vi "BioFeedback8(8-channelSubViewTo2DVR).vi"(0 "UI Data Right":path=path "C:/Users/Tinggroup/Desktop/VRMuscleActivationVisualizer/VRBiofeedback_v2/assets/RightEMGData.txt", 7 "Frames Per Second":dbl=30.0, 9 "Start Trial":bool, 11 "End Trial":bool, 12 "Data Directory":path, 13 "File Name":string, 14 "Extension":string="_EMG.txt") -> ()   [LabVIEW 2016]
uses:
  <vilib>/Utility/error.llb/DialogType.ctl
  <vilib>/Analysis/5stat.llb/RMS (DBL).vi
  <vilib>/Waveform/WDTOps.llb/WDT Append Waveforms DBL.vi
  <vilib>/Waveform/WDTFileIO.llb/Export Waveform To Spreadsheet File.vi
  <vilib>/Analysis/NI_AALPro.lvlib
panel:
  in  "UI Ampl Error Path":path=path "C:/Users/Tinggroup/Desktop/VRMuscleActivationVisualizer/VRBiofeedback_v2/assets/BiofeedbackAmplitudeError.txt"
  in  "UI L/R Error Path":path=path "C:/Users/Tinggroup/Desktop/VRMuscleActivationVisualizer/VRBiofeedback_v2/assets/BiofeedbackLRError.txt"
  out "LeftPercentActivation":dbl
  out "RightPercentActivation":dbl
  out "LeftMovingAvg":dbl
  out "RightMovingAvg":dbl
  out "Stability Data":dbl[](array[numeric])
  in  "StabilityBufferFramesCount":dbl=1.0
  out "StabilityFramesCount":dbl
  in  "GuageStability":bool
  out "StdDev":dbl
  out "Mean":dbl
  out "Min":dbl
  out "Max":dbl
  in  "AutoAnalyzeStablity":bool
  out "RMS Left Single Bucket":dbl(graph)
  out "PointCluster":cluster{dbl[], dbl[]}
  out "combined y value":dbl
  out "Acquiring Max":bool
  in  "endGetMax":bool
  in  "startGetMax":bool
  in  "Right Max":dbl
  in  "Left Max":dbl
  in  "Amplitude Error":dbl
  in  "L/R error":dbl
  out "Target Graph":cluster{dbl[], dbl[]}[](graph)
  in  "RightSignalB":dbl=6.0
  in  "RightSignalA":dbl=5.0
  in  "LefftSignalB":dbl=2.0
  in  "LeftSignalA":dbl=1.0
  out "Aggregate 8":waveform(dbl)[](array[waveform])
  in  "UI Data Left":path=path "C:/Users/Tinggroup/Desktop/VRMuscleActivationVisualizer/VRBiofeedback_v2/assets/LeftEMGData.txt"
  in  "EMG Input Device\nProduct Type":string="USB-6009"
  out "DispLeftMovingAvg":dbl(slide) max=1.0 scale=0.0..100.0
  out "DispRightMovingAvg":dbl(slide) max=0.01 scale=0.0..100.0
  out "RMS Right":dbl(graph)
  out "RMS Left":dbl(graph)
  out "RMS 8":dbl(graph)
  out "RMS 7":dbl(graph)
  out "RMS 6":dbl(graph)
  out "RMS 5":dbl(graph)
  out "RMS 4":dbl(graph)
  out "RMS 3":dbl(graph)
  out "RMS 2":dbl(graph)
  out "RMS 1":dbl(graph)
  out "Aggregate7":waveform(dbl)[](array[waveform])
  out "Aggregate6":waveform(dbl)[](array[waveform])
  out "Aggregate5":waveform(dbl)[](array[waveform])
  out "Aggregate4":waveform(dbl)[](array[waveform])
  out "Aggregate3":waveform(dbl)[](array[waveform])
  out "Aggregate2":waveform(dbl)[](array[waveform])
  out "Aggregate1":waveform(dbl)[](array[waveform])
  out "Wfm8":waveform(dbl)(graph)
  out "Wfm7":waveform(dbl)(graph)
  out "Wfm6":waveform(dbl)(graph)
  out "Wfm5":waveform(dbl)(graph)
  out "Wfm4":waveform(dbl)(graph)
  out "Wfm3":waveform(dbl)(graph)
  out "Wfm2":waveform(dbl)(graph)
  out "Wfm1":waveform(dbl)(graph)
  out "Trial Data":waveform(dbl)(graph)
  in  "UI Percent Path":path=path "C:/Users/Tinggroup/Desktop/VRMuscleActivationVisualizer/VRBiofeedback_v2/assets/BiofeedbackTargetPercentage.txt"
  in  "Target Percentage":dbl=10.0
  out "Trial In Progress":bool
  in  "Trial Number":dbl
  in  "MARK":bool
  in  "Lower Cut-Off":dbl=20.0
  in  "Upper Cut-Off":dbl=300.0
  out "raw data":dynamicdata(graph)
  out "Bufffer Index":dbl
  out "Frames in Buffer":dbl
  out "Samples per frame":dbl
  out "Reset Data Acquisition\nAnd UI Updating":bool=TRUE
  in  "Moving Average Length (s)":dbl=0.5
  in  "Sample rate (Hz)":dbl=2000.0
  in  "End Program":bool
  # "These \nSet \nThe \nTarget\nBox Size"
  # "Save Trial Data"
  # "These scale\nthe thermometers\nand are used in\nmean calculation"
  # "Auto Analyze Stability begins calculating stability\nAs soon as dot enters the target zone and stops \nonce the dot leaves the target zone"
  # "for testing smaller sample\nsizes in getting max/min\nand stability data"
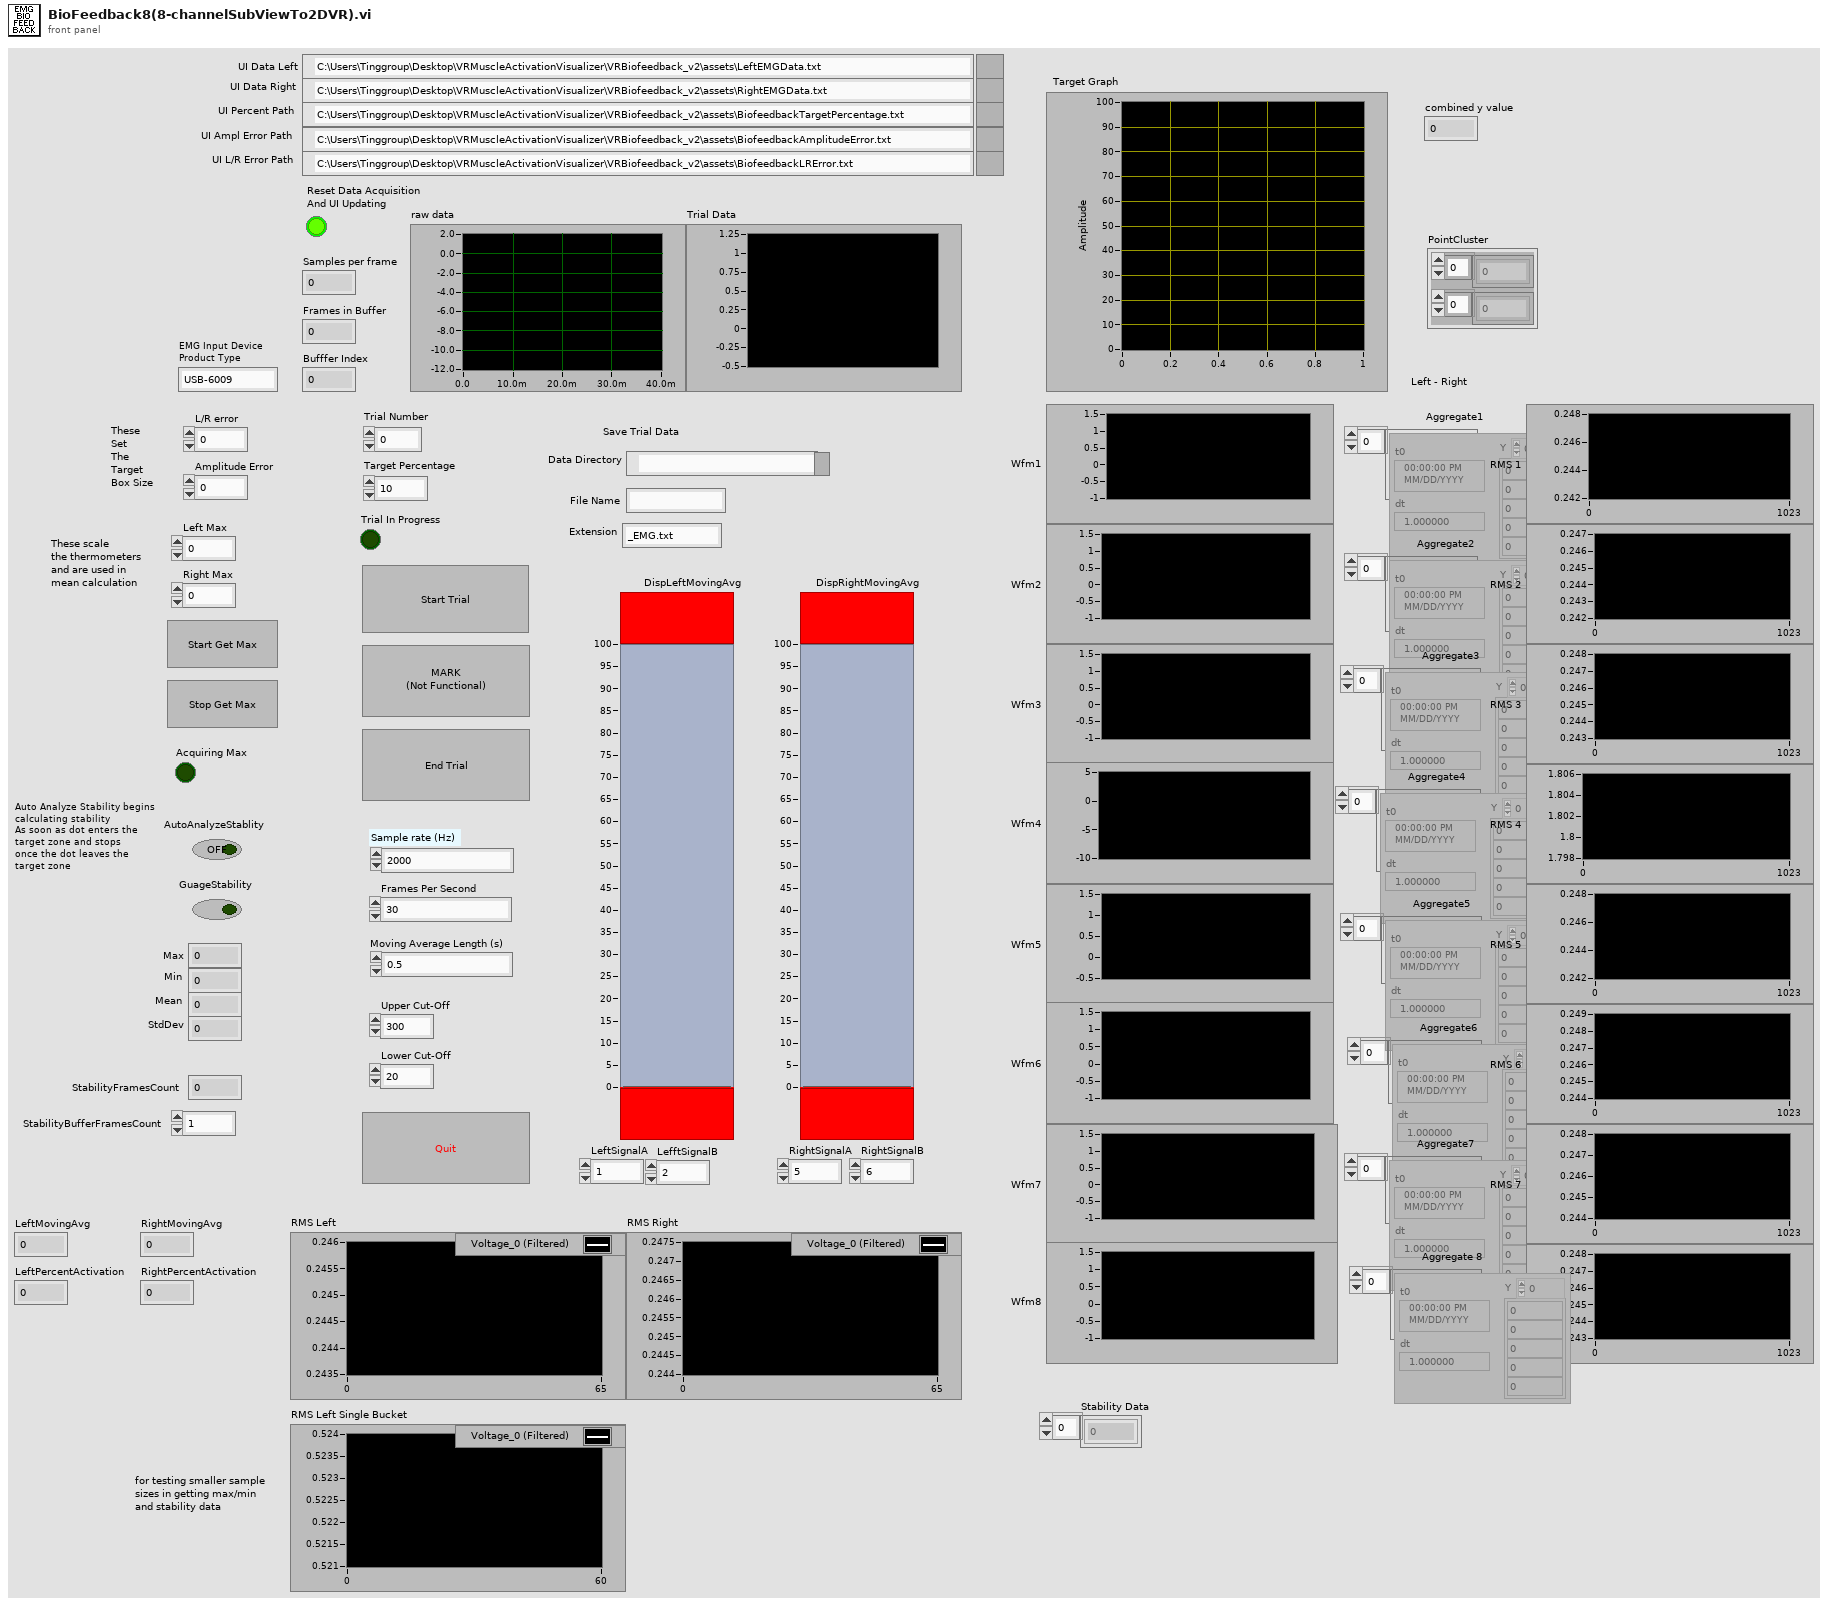
[diagram p1: front panel]
types:
  T1 = typedef "DialogType.ctl" = u16
  T2 = typedef "WaveformArrayControl.ctl" = waveform(dbl)[]
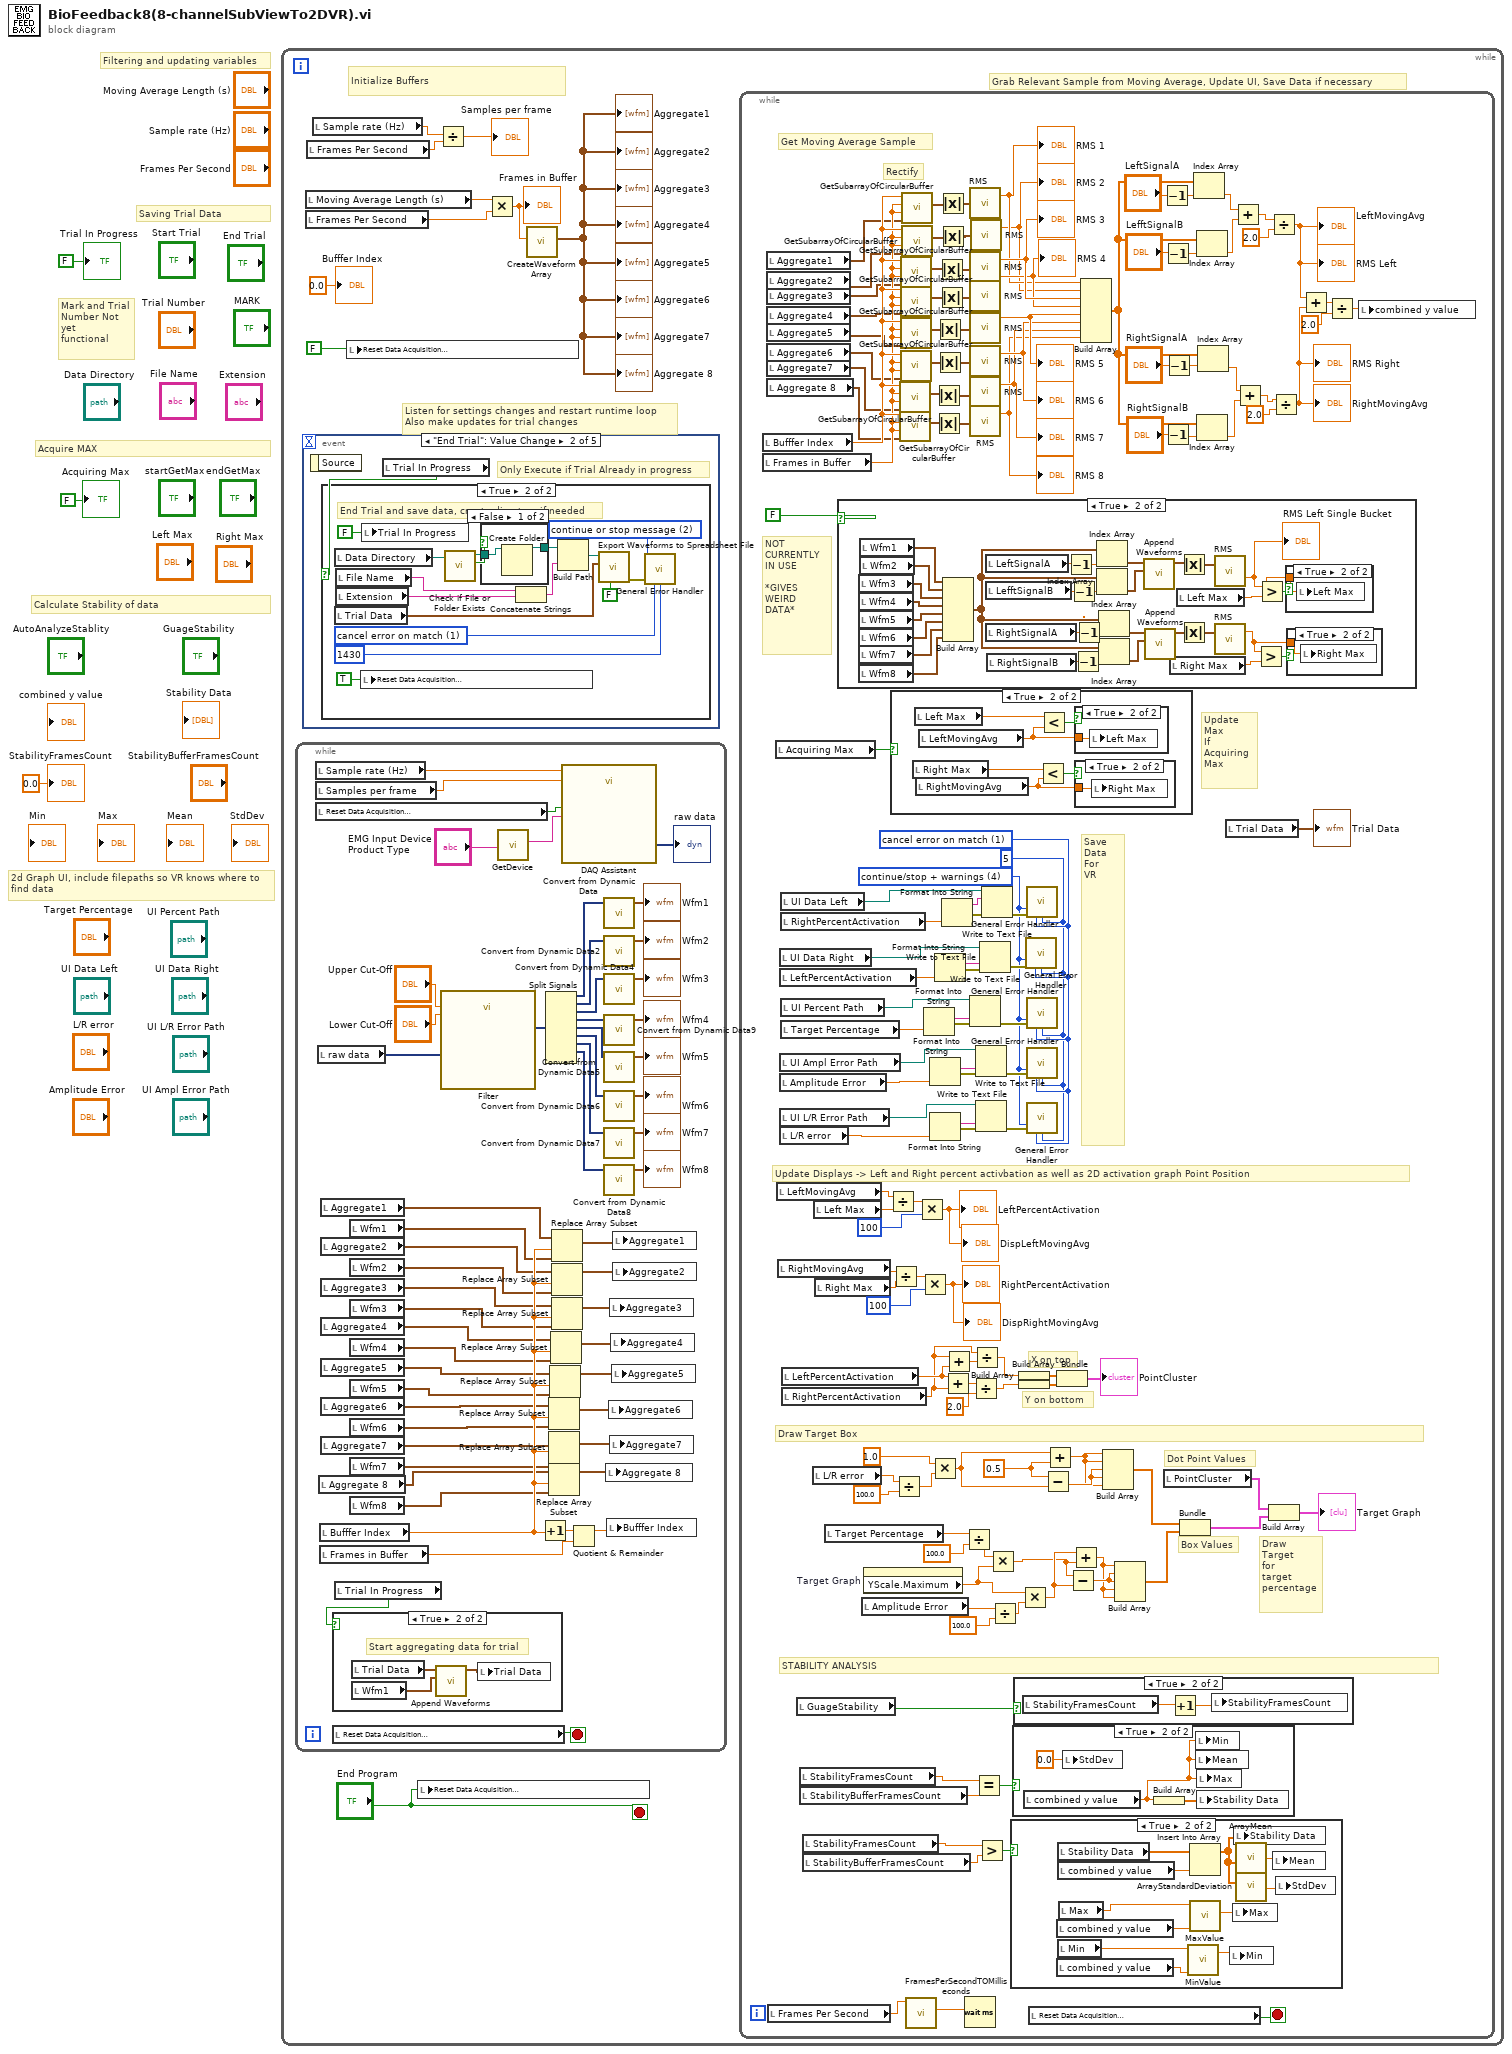
[diagram p0: block diagram]
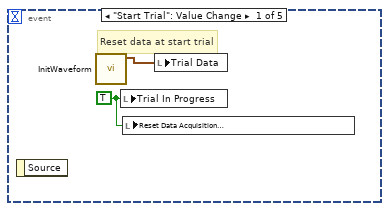
[diagram p2: hidden frame]
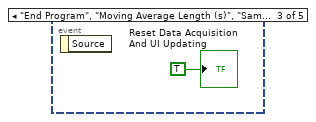
[diagram p5: hidden frame]
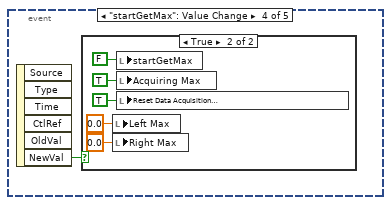
[diagram p6: hidden frame]
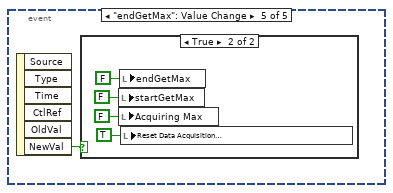
[diagram p8: hidden frame]
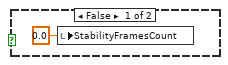
[diagram p12: hidden frame]
diagram:
  # "Calculate Stability of data"
  # "Acquire MAX"
  # "Filtering and updating variables"
  # "Saving Trial Data"
  # "2d Graph UI, include filepaths so VR knows where to find data"
  # "Mark and Trial Number Not yet \nfunctional"
  n1 = while {
    stop <- "End Program" stop-if-true
    # "Grab Relevant Sample from Moving Average, Update UI, Save Data if necessary"
    # "Initialize Buffers"
    # "Listen for settings changes and restart runtime loop\nAlso make updates for trial changes"
    n2 = while {
      stop <- w294 stop-if-true
      n3 = local read "Sample rate (Hz)"() -> (w302:dbl)
      n4 = local read "Samples per frame"() -> (w301:dbl)
      n5 = local read "Reset Data Acquisition\nAnd UI Updating"() -> (w293:bool)
      n6 = local read "raw data"() -> (w299:dynamicdata)
      n7 = local read "Aggregate 8"() -> (w249:waveform(dbl)[])
      n8 = local read "Bufffer Index"() -> (w274:dbl)
      n9 = local read "Frames in Buffer"() -> (w296:dbl)
      n10 = local read "Aggregate1"() -> (w273:waveform(dbl)[])
      n11 = local read "Aggregate2"() -> (w271:waveform(dbl)[])
      n12 = local read "Aggregate3"() -> (w269:waveform(dbl)[])
      n13 = local read "Aggregate4"() -> (w267:waveform(dbl)[])
      n14 = local read "Aggregate5"() -> (w265:waveform(dbl)[])
      n15 = local read "Aggregate6"() -> (w263:waveform(dbl)[])
      n16 = local read "Aggregate7"() -> (w261:waveform(dbl)[])
      n17 = local read "Reset Data Acquisition\nAnd UI Updating"() -> (w294:bool)
      n18 = local read "Trial In Progress"() -> (w251:bool)
      n19 = case shown="True" w251 {
        frame False {
        }
        frame True {
          # "Start aggregating data for trial"
          n20 = local read "Trial Data"() -> (w305:waveform(dbl))
          n21 = local read "Wfm1"() -> (w304:waveform(dbl))
          n22 = call-poly <vilib>:"Append Waveforms.vi"("waveform B"=w304, "waveform A"=w305) -> ("waveform out"=w303:waveform(dbl))  [unwired: 8 in, 1 out]
          n23 = local write "Trial Data"(w303) -> ()
        }
      }
      n24 = local read "Wfm1"() -> (w272:waveform(dbl))
      n25 = local read "Wfm2"() -> (w270:waveform(dbl))
      n26 = local read "Wfm3"() -> (w268:waveform(dbl))
      n27 = local read "Wfm4"() -> (w266:waveform(dbl))
      n28 = local read "Wfm5"() -> (w264:waveform(dbl))
      n29 = local read "Wfm6"() -> (w262:waveform(dbl))
      n30 = local read "Wfm7"() -> (w260:waveform(dbl))
      n31 = local read "Wfm8"() -> (w259:waveform(dbl))
      n32 = call "Filter"("Lower Cut-Off"="Lower Cut-Off", "Upper Cut-Off"="Upper Cut-Off", "Signal"=w299) -> ("Filtered Signal"=w291:dynamicdata)  [unwired: 7 in, 1 out]
      n33 = call "GetDevice.vi"("EMG Input Device\nProduct Type"="EMG Input Device\nProduct Type") -> ("DAQmx Device Name"=w247:tag)  [unwired: 10 in]
      n34 = Increment(x=w274) -> (x+1=w295:dbl)
      n35 = Split Signals(w291) -> (w290:dynamicdata, w289:dynamicdata, w288:dynamicdata, w287:dynamicdata, w286:dynamicdata, w285:dynamicdata, w284:dynamicdata, w283:dynamicdata)  [unwired: 9 in, 1 out]
      n36 = Replace Array Subset(array=w263, new element=w262, index=w274) -> (w253:waveform(dbl)[])
      n37 = Replace Array Subset(array=w261, new element=w260, index=w274) -> (w252:waveform(dbl)[])
      n38 = Replace Array Subset(array=w249, new element=w259, index=w274) -> (w250:waveform(dbl)[])
      n39 = Replace Array Subset(array=w265, new element=w264, index=w274) -> (w254:waveform(dbl)[])
      n40 = Replace Array Subset(array=w267, new element=w266, index=w274) -> (w255:waveform(dbl)[])
      n41 = Replace Array Subset(array=w273, new element=w272, index=w274) -> (w258:waveform(dbl)[])
      n42 = Replace Array Subset(array=w271, new element=w270, index=w274) -> (w257:waveform(dbl)[])
      n43 = Replace Array Subset(array=w269, new element=w268, index=w274) -> (w256:waveform(dbl)[])
      n44 = call "DAQ Assistant"("rate"=w302, "number of samples"=w301, "stop (T)"=w293, "device name"=w247) -> ("data"=→"raw data":dynamicdata)  [unwired: 13 in, 2 out]
      n45 = Quotient & Remainder(x=w295, y=w296) -> (x-y*floor(x/y)=w297:dbl)  [unwired: 1 out]
      n46 = call "Convert from Dynamic Data"("Dynamic Data Type"=w290) -> ("Waveform"=→"Wfm1":waveform(dbl))  [unwired: 3 in]
      n47 = call "Convert from Dynamic Data2"("Dynamic Data Type"=w289) -> ("Waveform"=→"Wfm2":waveform(dbl))  [unwired: 3 in]
      n48 = call "Convert from Dynamic Data4"("Dynamic Data Type"=w288) -> ("Waveform"=→"Wfm3":waveform(dbl))  [unwired: 3 in]
      n49 = call "Convert from Dynamic Data9"("Dynamic Data Type"=w287) -> ("Waveform"=→"Wfm4":waveform(dbl))  [unwired: 3 in]
      n50 = call "Convert from Dynamic Data5"("Dynamic Data Type"=w286) -> ("Waveform"=→"Wfm5":waveform(dbl))  [unwired: 3 in]
      n51 = call "Convert from Dynamic Data6"("Dynamic Data Type"=w285) -> ("Waveform"=→"Wfm6":waveform(dbl))  [unwired: 3 in]
      n52 = call "Convert from Dynamic Data7"("Dynamic Data Type"=w284) -> ("Waveform"=→"Wfm7":waveform(dbl))  [unwired: 3 in]
      n53 = call "Convert from Dynamic Data8"("Dynamic Data Type"=w283) -> ("Waveform"=→"Wfm8":waveform(dbl))  [unwired: 3 in]
      n54 = local write "Aggregate 8"(w250) -> ()
      n55 = local write "Bufffer Index"(w297) -> ()
      n56 = local write "Aggregate6"(w253) -> ()
      n57 = local write "Aggregate3"(w256) -> ()
      n58 = local write "Aggregate7"(w252) -> ()
      n59 = local write "Aggregate4"(w255) -> ()
      n60 = local write "Aggregate5"(w254) -> ()
      n61 = local write "Aggregate1"(w258) -> ()
      n62 = local write "Aggregate2"(w257) -> ()
    }
    n63 = event shown="[1] \"End Trial\": Value Change" {
      selector: _ -> [_ _ _ _ _]
      dyn-events: _ -> [_ _ _ _ _]
      timeout: _ -> [_ _ _ _ _]
      event "Start Trial": Value Change {
        w14 = TRUE ("Trial In Progress")
        # "Reset data at start trial"
        n64 = event-data() -> ()  [unwired: 1 in, 1 out]
        n65 = call "InitWaveform.vi"() -> ("output waveform"=w15:waveform(dbl))  [unwired: 11 in]
        n66 = local write "Trial In Progress"(w14) -> ()
        n67 = local write "Reset Data Acquisition\nAnd UI Updating"(w14) -> ()
        n68 = local write "Trial Data"(w15) -> ()
      }
      event "End Trial": Value Change {
        # "Only Execute if Trial Already in progress"
        n69 = event-data() -> ()  [unwired: 1 in, 1 out]
        n70 = local read "Trial In Progress"() -> (w16:bool)
        n71 = case shown="True" w16 {
          frame False {
          }
          frame True {
            w25 = T1 2 items=["no dialog", "OK message", "continue or stop message", "OK message + warnings", "continue/stop + warnings"] ("type of dialog (OK msg:1)")
            w26 = 1 items=["no exception", "cancel error on match", "set error on match"] ("[exception action] (none:0)")
            # "End Trial and save data, create directory if needed"
            n72 = local read "Data Directory"() -> (w28:path)
            n73 = local read "Trial Data"() -> (w18:waveform(dbl))
            n74 = local read "File Name"() -> (w20:string)
            n75 = local read "Extension"() -> (w21:string)
            n76 = local write "Reset Data Acquisition\nAnd UI Updating"(TRUE ("Reset Data Acquisition\nAnd UI Updating")) -> ()
            n77 = local write "Trial In Progress"(FALSE ("Trial In Progress")) -> ()
            n78 = call <vilib>:"Check if File or Folder Exists.vi"("path"=w28) -> ("file or folder exists?"=w30:bool, "dup path"=w29:path)  [unwired: 8 in, 1 out]
            n79 = case shown="False" w30 {
              tunnel: [w33 w35] -> w24
              tunnel: w29 -> [w34 w35]
              frame False {
                n80 = Create Folder(path (use dialog)=w34) -> (created path=w33:path)  [unwired: 2 in, 2 out]
              }
              frame True {
              }
            }
            n81 = Concatenate Strings(w20, w21) -> (w19:string)
            n82 = Build Path(base path=w24, name or relative path=w19) -> (appended path=w23:path)
            n83 = call-poly <vilib>:"Export Waveforms to Spreadsheet File.vi"("append to file? (new file:F)"=FALSE, "waveform"=w18, "file path (dialog if empty)"=w23) -> ("error out"=w17:errorcluster)  [unwired: 7 in, 1 out]
            n84 = call <vilib>:"General Error Handler.vi"("type of dialog (OK msg:1)"=w25, "error in (no error)"=w17, "[exception action] (none:0)"=w26, "[exception code]"=1430) -> ()  [unwired: 7 in, 5 out]
          }
        }
      }
      event "End Program", "Moving Average Length (s)", "Sample rate (Hz)", "Frames Per Second": Value Change {
        n85 = event-data() -> ()  [unwired: 1 in, 1 out]
        "Reset Data Acquisition\nAnd UI Updating" <- TRUE
      }
      event "startGetMax": Value Change {
        n86 = event-data() -> ("NewVal"=w37:bool)  [unwired: 1 in, 5 out]
        n87 = case shown="True" w37 {
          frame False {
          }
          frame True {
            n88 = local write "Left Max"(0.0 ("Left Max")) -> ()
            n89 = local write "Right Max"(0.0 ("Right Max")) -> ()
            n90 = local write "startGetMax"(FALSE) -> ()
            n91 = local write "Acquiring Max"(TRUE ("Acquiring Max")) -> ()
            n92 = local write "Reset Data Acquisition\nAnd UI Updating"(TRUE ("Reset Data Acquisition\nAnd UI Updating")) -> ()
          }
        }
      }
      event "endGetMax": Value Change {
        n93 = event-data() -> ("NewVal"=w43:bool)  [unwired: 1 in, 5 out]
        n94 = case shown="True" w43 {
          frame False {
          }
          frame True {
            n95 = local write "startGetMax"(FALSE ("startGetMax")) -> ()
            n96 = local write "Acquiring Max"(FALSE ("Acquiring Max")) -> ()
            n97 = local write "endGetMax"(FALSE ("endGetMax")) -> ()
            n98 = local write "Reset Data Acquisition\nAnd UI Updating"(TRUE ("Reset Data Acquisition\nAnd UI Updating")) -> ()
          }
        }
      }
    }
    n99 = local read "Moving Average Length (s)"() -> (w10:dbl)
    n100 = local read "Frames Per Second"() -> (w9:dbl)
    n101 = local read "Frames Per Second"() -> (w12:dbl)
    n102 = local read "Sample rate (Hz)"() -> (w13:dbl)
    n103 = local write "Reset Data Acquisition\nAnd UI Updating"(FALSE) -> ()
    n104 = local write "Reset Data Acquisition\nAnd UI Updating"("End Program") -> ()
    n105 = Divide(x=w13, y=w12) -> (x/y=→"Samples per frame":dbl)
    n106 = Multiply(x=w10, y=w9) -> (x*y=w6:dbl)
    "Frames in Buffer" <- w6
    n107 = call "CreateWaveformArray.vi"("bufferSize"=w6) -> ("initialized array"=→"Aggregate1" →"Aggregate2" →"Aggregate3" →"Aggregate4" →"Aggregate5" →"Aggregate6" →"Aggregate7" →"Aggregate 8":waveform(dbl)[])  [unwired: 5 in, 1 out]
    n108 = while {
      stop <- w188 stop-if-true
      w106 = 0.5 ("element")
      w50 = T1 4 items=["no dialog", "OK message", "continue or stop message", "OK message + warnings", "continue/stop + warnings"] ("type of dialog (OK msg:1)")
      w49 = 1 items=["no exception", "cancel error on match", "set error on match"] ("[exception action] (none:0)")
      w48 = 5 ("[exception code]")
      # "Y on bottom"
      # "X on top"
      # "Dot Point Values"
      # "Box Values"
      # "Update Displays -> Left and Right percent activbation as well as 2D activation graph Point Position"
      # "STABILITY ANALYSIS"
      # "NOT\nCURRENTLY\nIN USE\n\n*GIVES\nWEIRD\nDATA*"
      # "Draw \nTarget\nfor\ntarget\npercentage"
      # "Draw Target Box"
      # "Update\nMax\nIf \nAcquiring\nMax"
      # "Save\nData\nFor\nVR"
      # "Get Moving Average Sample"
      # "Rectify"
      n109 = local read "Bufffer Index"() -> (w179:dbl)
      n110 = local read "Frames in Buffer"() -> (w178:dbl)
      n111 = local read "Aggregate1"() -> (w177:waveform(dbl)[])
      n112 = local read "Aggregate2"() -> (w173:waveform(dbl)[])
      n113 = local read "Aggregate3"() -> (w176:waveform(dbl)[])
      n114 = local read "Aggregate4"() -> (w172:waveform(dbl)[])
      n115 = local read "Aggregate5"() -> (w175:waveform(dbl)[])
      n116 = local read "Aggregate6"() -> (w174:waveform(dbl)[])
      n117 = local read "Aggregate7"() -> (w171:waveform(dbl)[])
      n118 = local read "Aggregate 8"() -> (w145:waveform(dbl)[])
      n119 = local read "Frames Per Second"() -> (w187:dbl)
      n120 = local read "Acquiring Max"() -> (w90:bool)
      n121 = local read "LeftMovingAvg"() -> (w79:dbl)
      n122 = local read "RightMovingAvg"() -> (w75:dbl)
      n123 = local read "UI Data Right"() -> (w183:path)
      n124 = local read "LeftPercentActivation"() -> (w181:dbl)
      n125 = local read "UI Ampl Error Path"() -> (w51:path)
      n126 = local read "Amplitude Error"() -> (w52:dbl)
      n127 = local read "UI L/R Error Path"() -> (w54:path)
      n128 = local read "L/R error"() -> (w53:dbl)
      n129 = local read "UI Data Left"() -> (w153:path)
      n130 = local read "RightPercentActivation"() -> (w155:dbl)
      n131 = local read "UI Percent Path"() -> (w147:path)
      n132 = local read "Target Percentage"() -> (w146:dbl)
      n133 = local read "LeftPercentActivation"() -> (w68:dbl)
      n134 = local read "RightPercentActivation"() -> (w66:dbl)
      n135 = local read "GuageStability"() -> (w88:bool)
      n136 = local read "StabilityFramesCount"() -> (w87:dbl)
      n137 = local read "StabilityBufferFramesCount"() -> (w86:dbl)
      n138 = local read "StabilityFramesCount"() -> (w84:dbl)
      n139 = local read "StabilityBufferFramesCount"() -> (w83:dbl)
      n140 = local read "L/R error"() -> (w125:dbl)
      n141 = local read "Left Max"() -> (w78:dbl)
      n142 = local read "Right Max"() -> (w74:dbl)
      n143 = local read "Target Percentage"() -> (w122:dbl)
      n144 = case shown="True" FALSE {
        frame False {
        }
        frame True {
          n145 = local read "Wfm3"() -> (w237:waveform(dbl))
          n146 = local read "Wfm4"() -> (w236:waveform(dbl))
          n147 = local read "Wfm5"() -> (w240:waveform(dbl))
          n148 = local read "Wfm6"() -> (w241:waveform(dbl))
          n149 = local read "Wfm7"() -> (w242:waveform(dbl))
          n150 = local read "Wfm8"() -> (w243:waveform(dbl))
          n151 = local read "Wfm1"() -> (w239:waveform(dbl))
          n152 = local read "Wfm2"() -> (w238:waveform(dbl))
          n153 = Build Array(w239, w238, w237, w236, w240, w241, w242, w243) -> (w235:waveform(dbl)[])
          n154 = local read "LeftSignalA"() -> (w221:dbl)
          n155 = local read "LefftSignalB"() -> (w219:dbl)
          n156 = local read "RightSignalA"() -> (w217:dbl)
          n157 = local read "RightSignalB"() -> (w214:dbl)
          n158 = Decrement(x=w221) -> (x-1=w220:dbl)
          n159 = Decrement(x=w219) -> (x-1=w218:dbl)
          n160 = Decrement(x=w214) -> (x-1=w215:dbl)
          n161 = Decrement(x=w217) -> (x-1=w216:dbl)
          n162 = Index Array(array=w235, index=w220) -> (element=w222:waveform(dbl))
          n163 = Index Array(array=w235, index=w218) -> (element=w223:waveform(dbl))
          n164 = Index Array(array=w235, index=w216) -> (element=w234:waveform(dbl))
          n165 = Index Array(array=w235, index=w215) -> (element=w233:waveform(dbl))
          n166 = call-poly <vilib>:"Append Waveforms.vi"("waveform B"=w223, "waveform A"=w222) -> ("waveform out"=w229:waveform(dbl))  [unwired: 8 in, 1 out]
          n167 = call-poly <vilib>:"Append Waveforms.vi"("waveform B"=w233, "waveform A"=w234) -> ("waveform out"=w232:waveform(dbl))  [unwired: 8 in, 1 out]
          n168 = local read "Right Max"() -> (w228:dbl)
          n169 = local read "Left Max"() -> (w244:dbl)
          n170 = Absolute Value(x=w229) -> (abs(x)=w230:waveform(dbl))
          n171 = Absolute Value(x=w232) -> (abs(x)=w231:waveform(dbl))
          n172 = call-poly <vilib>:"RMS.vi"("X"=w230) -> ("rms value"=w224:dbl)  [unwired: 1 out]
          "RMS Left Single Bucket" <- w224
          n173 = call-poly <vilib>:"RMS.vi"("X"=w231) -> ("rms value"=w227:dbl)  [unwired: 1 out]
          n174 = Greater?(x=w227, y=w228) -> (0:w226:bool)
          n175 = Greater?(x=w224, y=w244) -> (0:w225:bool)
          n176 = case shown="True" w225 {
            tunnel: w224 -> [_ w246]
            frame False {
            }
            frame True {
              n177 = local write "Left Max"(w246) -> ()
            }
          }
          n178 = case shown="True" w226 {
            tunnel: w227 -> [_ w245]
            frame False {
            }
            frame True {
              n179 = local write "Right Max"(w245) -> ()
            }
          }
        }
      }
      n180 = local read "Amplitude Error"() -> (w124:dbl)
      n181 = property on="Target Graph" class="XYGraph (strict)"() -> ("YScale.Maximum"=w104:dbl)  [unwired: 2 in, 2 out]
      n182 = Divide(x=w79, y=w78) -> (x/y=w80:dbl)
      n183 = case shown="True" w90 {
        frame False {
        }
        frame True {
          n184 = local read "Right Max"() -> (w208:dbl)
          n185 = local read "Left Max"() -> (w211:dbl)
          n186 = local read "RightMovingAvg"() -> (w206:dbl)
          n187 = local read "LeftMovingAvg"() -> (w210:dbl)
          n188 = Less?(x=w208, y=w206) -> (x < y?=w207:bool)
          n189 = Less?(x=w211, y=w210) -> (x < y?=w209:bool)
          n190 = case shown="True" w209 {
            tunnel: w210 -> [_ w213]
            frame False {
            }
            frame True {
              n191 = local write "Left Max"(w213) -> ()
            }
          }
          n192 = case shown="True" w207 {
            tunnel: w206 -> [_ w212]
            frame False {
            }
            frame True {
              n193 = local write "Right Max"(w212) -> ()
            }
          }
        }
      }
      n194 = Divide(x=w75, y=w74) -> (x/y=w76:dbl)
      n195 = Divide(x=w125, y=100.0) -> (x/y=w114:dbl)
      n196 = call "GetSubarrayOfCircularBuffer.vi"("initialized array"=w171, "buffer size"=w178, "subset size"=w178, "start index"=w179) -> ("initialized array 2"=w164:T2)  [unwired: 7 in]
      n197 = call "GetSubarrayOfCircularBuffer.vi"("initialized array"=w145, "buffer size"=w178, "subset size"=w178, "start index"=w179) -> ("initialized array 2"=w163:T2)  [unwired: 7 in]
      n198 = call "GetSubarrayOfCircularBuffer.vi"("initialized array"=w176, "buffer size"=w178, "subset size"=w178, "start index"=w179) -> ("initialized array 2"=w168:T2)  [unwired: 7 in]
      n199 = call "GetSubarrayOfCircularBuffer.vi"("initialized array"=w172, "buffer size"=w178, "subset size"=w178, "start index"=w179) -> ("initialized array 2"=w167:T2)  [unwired: 7 in]
      n200 = call "GetSubarrayOfCircularBuffer.vi"("initialized array"=w175, "buffer size"=w178, "subset size"=w178, "start index"=w179) -> ("initialized array 2"=w166:T2)  [unwired: 7 in]
      n201 = call "GetSubarrayOfCircularBuffer.vi"("initialized array"=w174, "buffer size"=w178, "subset size"=w178, "start index"=w179) -> ("initialized array 2"=w165:T2)  [unwired: 7 in]
      n202 = call "GetSubarrayOfCircularBuffer.vi"("initialized array"=w177, "buffer size"=w178, "subset size"=w178, "start index"=w179) -> ("initialized array 2"=w170:T2)  [unwired: 7 in]
      n203 = call "GetSubarrayOfCircularBuffer.vi"("initialized array"=w173, "buffer size"=w178, "subset size"=w178, "start index"=w179) -> ("initialized array 2"=w169:T2)  [unwired: 7 in]
      n204 = call "FramesPerSecondTOMilliseconds.vi"("Thermometer\nFps"=w187) -> ("x*y"=w186:dbl)  [unwired: 10 in]
      n205 = Multiply(x=w80, y=100) -> (x*y=→"DispLeftMovingAvg" →"LeftPercentActivation":dbl)
      n206 = Multiply(x=w76, y=100) -> (x*y=→"DispRightMovingAvg" →"RightPercentActivation":dbl)
      n207 = Format Into String(w146) -> (resulting string=w148:string, error out=w149:errorcluster)  [unwired: 3 in]
      n208 = Format Into String(w52) -> (resulting string=w58:string, error out=w59:errorcluster)  [unwired: 3 in]
      n209 = Format Into String(w53) -> (resulting string=w55:string, error out=w56:errorcluster)  [unwired: 3 in]
      n210 = Multiply(x=1.0, y=w114) -> (x*y=w113:dbl)
      n211 = Absolute Value(x=w164) -> (abs(x)=w157:T2)
      n212 = Absolute Value(x=w163) -> (abs(x)=w156:T2)
      n213 = Absolute Value(x=w166) -> (abs(x)=w159:T2)
      n214 = Absolute Value(x=w165) -> (abs(x)=w158:T2)
      n215 = Format Into String(w181) -> (resulting string=w182:string, error out=w184:errorcluster)  [unwired: 3 in]
      n216 = Absolute Value(x=w168) -> (abs(x)=w161:T2)
      n217 = Absolute Value(x=w167) -> (abs(x)=w160:T2)
      n218 = Absolute Value(x=w170) -> (abs(x)=w162:T2)
      n219 = Absolute Value(x=w169) -> (abs(x)=w144:T2)
      n220 = Format Into String(w155) -> (resulting string=w152:string, error out=w154:errorcluster)  [unwired: 3 in]
      n221 = Add(x=w68, y=w66) -> (x+y=w70:dbl)
      n222 = Add(x=w66, y=w68) -> (x+y=w67:dbl)
      n223 = Divide(x=w122, y=100.0) -> (x/y=w105:dbl)
      n224 = Wait (ms)(milliseconds to wait=w186) -> ()  [unwired: 1 out]
      n225 = call-poly <vilib>:"RMS.vi"("X"=w162) -> ("rms value"=w138:dbl)  [unwired: 1 out]
      "RMS 1" <- w138
      n226 = call-poly <vilib>:"RMS.vi"("X"=w161) -> ("rms value"=w143:dbl)  [unwired: 1 out]
      "RMS 3" <- w143
      n227 = call-poly <vilib>:"RMS.vi"("X"=w160) -> ("rms value"=w142:dbl)  [unwired: 1 out]
      "RMS 4" <- w142
      n228 = call-poly <vilib>:"RMS.vi"("X"=w159) -> ("rms value"=w141:dbl)  [unwired: 1 out]
      "RMS 5" <- w141
      n229 = call-poly <vilib>:"RMS.vi"("X"=w158) -> ("rms value"=w140:dbl)  [unwired: 1 out]
      "RMS 6" <- w140
      n230 = call-poly <vilib>:"RMS.vi"("X"=w157) -> ("rms value"=w139:dbl)  [unwired: 1 out]
      "RMS 7" <- w139
      n231 = call-poly <vilib>:"RMS.vi"("X"=w156) -> ("rms value"=w136:dbl)  [unwired: 1 out]
      "RMS 8" <- w136
      n232 = Write to Text File(file (use dialog)=w147, text=w148, error in=w149) -> (error out=w150:errorcluster)  [unwired: 1 in, 2 out]
      n233 = call-poly <vilib>:"RMS.vi"("X"=w144) -> ("rms value"=w137:dbl)  [unwired: 1 out]
      "RMS 2" <- w137
      n234 = Divide(x=w70, y=2.0) -> (x/y=w69:dbl)
      n235 = Divide(x=w66, y=w67) -> (x/y=w65:dbl)
      n236 = Equal?(x=w87, y=w86) -> (x = y?=w85:bool)
      n237 = Write to Text File(file (use dialog)=w51, text=w58, error in=w59) -> (error out=w60:errorcluster)  [unwired: 1 in, 2 out]
      n238 = Write to Text File(file (use dialog)=w54, text=w55, error in=w56) -> (error out=w57:errorcluster)  [unwired: 1 in, 2 out]
      n239 = Greater?(x=w84, y=w83) -> (0:w82:bool)
      n240 = Write to Text File(file (use dialog)=w183, text=w182, error in=w184) -> (error out=w185:errorcluster)  [unwired: 1 in, 2 out]
      n241 = Write to Text File(file (use dialog)=w153, text=w152, error in=w154) -> (error out=w151:errorcluster)  [unwired: 1 in, 2 out]
      n242 = Multiply(x=w105, y=w104) -> (x*y=w110:dbl)
      n243 = Divide(x=w124, y=100.0) -> (x/y=w112:dbl)
      n244 = case shown="True" w82 {
        frame False {
        }
        frame True {
          n245 = local read "combined y value"() -> (w197:dbl)
          n246 = local read "combined y value"() -> (w194:dbl)
          n247 = local read "Stability Data"() -> (w199:dbl[])
          n248 = local read "combined y value"() -> (w198:dbl)
          n249 = local read "Min"() -> (w195:dbl)
          n250 = local read "Max"() -> (w196:dbl)
          n251 = call "MinValue.vi"("CurrentMin"=w195, "NewValue"=w194) -> ("Min"=w193:dbl)  [unwired: 8 in]
          n252 = Insert Into Array(array=w199, new element=w198) -> (w189:dbl[])  [unwired: 1 in]
          n253 = call "MaxValue.vi"("NewValue"=w197, "CurrentMax"=w196) -> ("Max"=w192:dbl)  [unwired: 9 in]
          n254 = local write "Min"(w193) -> ()
          n255 = local write "Max"(w192) -> ()
          n256 = local write "Stability Data"(w189) -> ()
          n257 = call "ArrayMean.vi"("Array"=w189) -> ("Mean"=w191:dbl)  [unwired: 10 in]
          n258 = call "ArrayStandardDeviation.vi"("Array"=w189) -> ("StdDev"=w190:dbl)  [unwired: 10 in]
          n259 = local write "Mean"(w191) -> ()
          n260 = local write "StdDev"(w190) -> ()
        }
      }
      n261 = case shown="True" w85 {
        frame False {
        }
        frame True {
          n262 = local read "combined y value"() -> (w200:dbl)
          n263 = local write "StdDev"(0.0 ("StdDev")) -> ()
          n264 = Build Array(w200) -> (w201:dbl[])
          n265 = local write "Min"(w200) -> ()
          n266 = local write "Mean"(w200) -> ()
          n267 = local write "Max"(w200) -> ()
          n268 = local write "Stability Data"(w201) -> ()
        }
      }
      n269 = case shown="True" w88 {
        frame False {
          n270 = local write "StabilityFramesCount"(0.0 ("StabilityFramescount")) -> ()
        }
        frame True {
          n271 = local read "StabilityFramesCount"() -> (w205:dbl)
          n272 = Increment(x=w205) -> (x+1=w204:dbl)
          n273 = local write "StabilityFramesCount"(w204) -> ()
        }
      }
      n274 = Build Array(w65) -> (w130:dbl[])
      n275 = Build Array(w69) -> (w128:dbl[])
      n276 = Multiply(x=w104, y=w112) -> (x*y=w111:dbl)
      n277 = call <vilib>:"General Error Handler.vi"("type of dialog (OK msg:1)"=w50, "error in (no error)"=w185, "[exception action] (none:0)"=w49, "[exception code]"=w48) -> ()  [unwired: 7 in, 5 out]
      n278 = call <vilib>:"General Error Handler.vi"("type of dialog (OK msg:1)"=w50, "error in (no error)"=w151, "[exception action] (none:0)"=w49, "[exception code]"=w48) -> ()  [unwired: 7 in, 5 out]
      n279 = call <vilib>:"General Error Handler.vi"("type of dialog (OK msg:1)"=w50, "error in (no error)"=w150, "[exception action] (none:0)"=w49, "[exception code]"=w48) -> ()  [unwired: 7 in, 5 out]
      n280 = call <vilib>:"General Error Handler.vi"("type of dialog (OK msg:1)"=w50, "error in (no error)"=w60, "[exception action] (none:0)"=w49, "[exception code]"=w48) -> ()  [unwired: 7 in, 5 out]
      n281 = call <vilib>:"General Error Handler.vi"("type of dialog (OK msg:1)"=w50, "error in (no error)"=w57, "[exception action] (none:0)"=w49, "[exception code]"=w48) -> ()  [unwired: 7 in, 5 out]
      n282 = local read "Reset Data Acquisition\nAnd UI Updating"() -> (w188:bool)
      n283 = Subtract(x=w106, y=w113) -> (x-y=w120:dbl)
      n284 = Add(x=w113, y=w106) -> (x+y=w115:dbl)
      n285 = Bundle(w130, w128) -> (→"PointCluster":cluster{dbl[], dbl[]})  [unwired: 1 in]
      n286 = Subtract(x=w110, y=w111) -> (x-y=w117:dbl)
      n287 = Add(x=w111, y=w110) -> (x+y=w116:dbl)
      n288 = Build Array(w138, w137, w143, w142, w141, w140, w139, w136) -> (w135:dbl[])
      n289 = Build Array(w115, w115, w120, w120, w115) -> (w108:dbl[])
      n290 = Build Array(w116, w117, w117, w116, w116) -> (w109:dbl[])
      n291 = Decrement(x="LeftSignalA") -> (x-1=w95:dbl)
      n292 = Decrement(x="LefftSignalB") -> (x-1=w97:dbl)
      n293 = Decrement(x="RightSignalB") -> (x-1=w93:dbl)
      n294 = Decrement(x="RightSignalA") -> (x-1=w91:dbl)
      n295 = local read "PointCluster"() -> (w103:cluster{dbl[], dbl[]})
      n296 = Bundle(w108, w109) -> (w118:cluster{dbl[], dbl[]})  [unwired: 1 in]
      n297 = Index Array(array=w135, index=w95) -> (element=w102:dbl)
      n298 = Index Array(array=w135, index=w97) -> (element=w101:dbl)
      n299 = Index Array(array=w135, index=w93) -> (element=w133:dbl)
      n300 = Index Array(array=w135, index=w91) -> (element=w134:dbl)
      n301 = local read "Trial Data"() -> (→"Trial Data":waveform(dbl))
      n302 = Add(x=w102, y=w101) -> (x+y=w100:dbl)
      n303 = Add(x=w134, y=w133) -> (x+y=w131:dbl)
      n304 = Divide(x=w100, y=2.0) -> (x/y=w61:dbl)
      "RMS Left" <- w61
      "LeftMovingAvg" <- w61
      n305 = Build Array(w103, w118) -> (→"Target Graph":cluster{dbl[], dbl[]}[])
      n306 = Divide(x=w131, y=2.0) -> (x/y=w62:dbl)
      "RMS Right" <- w62
      "RightMovingAvg" <- w62
      n307 = Add(x=w61, y=w62) -> (x+y=w129:dbl)
      n308 = Divide(x=w129, y=2.0) -> (x/y=w127:dbl)
      n309 = local write "combined y value"(w127) -> ()
    }
    "Bufffer Index" <- 0.0 ("Bufffer Index")
  }
  "Trial In Progress" <- FALSE ("Trial In Progress")
  "Acquiring Max" <- FALSE ("Acquiring Max")
  "StabilityFramesCount" <- 0.0 ("StabilityFramescount")
